vi "YOLO11_OBB_OpenVINO_NIVision.vi"() -> ()   [LabVIEW 2018]
doc: "YOLO11_OBB_OpenVINO_NIVision: This example integrates the YOLO11 algorithm with OpenVINO for object detection with oriented bounding boxes (OBB), specifically using the NI Vision (NIVision) library for enhanced image processing. The combination leverages the power of OpenVINO for optimized inference across Intel hardware and the NI Vision library for advanced vision functions, such as image acquisition, processing, and analysis. The model detects objects in images or video streams and generates oriented bounding boxes (OBB) that provide both the position and rotation of each object, enabling precise localization of rotated or irregularly shaped items. This solution is ideal for real-time industrial or automation applications, where both detection accuracy and processing efficiency are critical. Through the use of OpenVINO and NIVision, the model can run on a variety of platforms, ensuring scalability and performance in diverse environments."
uses:
  vi.lib/VIRobotics/ModelZoo/Object_Detection/yolov8_obb_openvino/Initial_yolo11_Obb_OpenVINO.vi
  vi.lib/VIRobotics/ModelZoo/Object_Detection/yolov8_obb_openvino/yolov8_obb_openvino.lvclass
  <vilib>/vision/driver/NI_Vision_Acquisition_Software.lvlib
panel:
  in  "device_name":string(combo)="CPU"
  in  "class_names_file":path=path "C:/ProgramData/VIRobotics/ModelZoo/Object_Detection/coco.names"
  in  "model_file":path=path "C:/ProgramData/VIRobotics/ModelZoo/Object_Detection/yolo11_obb/onnx_model/yolo11n-obb.onnx"
  in  "Camera Name":refnum<k21>="cam0" caption="IMAQdx Session"
  out "Image":T1(plugin-control)
  in  "Stop":bool
  out "每帧耗时(s)":dbl
  # "Overview: Demonstrates how to use OpenVINO to load the the ONNX model of yolo11_obb for real-time object detection.\nRequirements: Windows.\nMake sure your computer has a camera。\nInstructions: \n1.Select the device_name to use.（If your computer has Intel GPU, you can select GPU in the \"type\" control before running the VI to achieve faster inference).\n2.Run the VI.\nIf you want to load the model you trained, follow the following steps:\n1.Select the device_name to use. \n2.Specify the model_file and class_names_file.\n3.Run the VI."
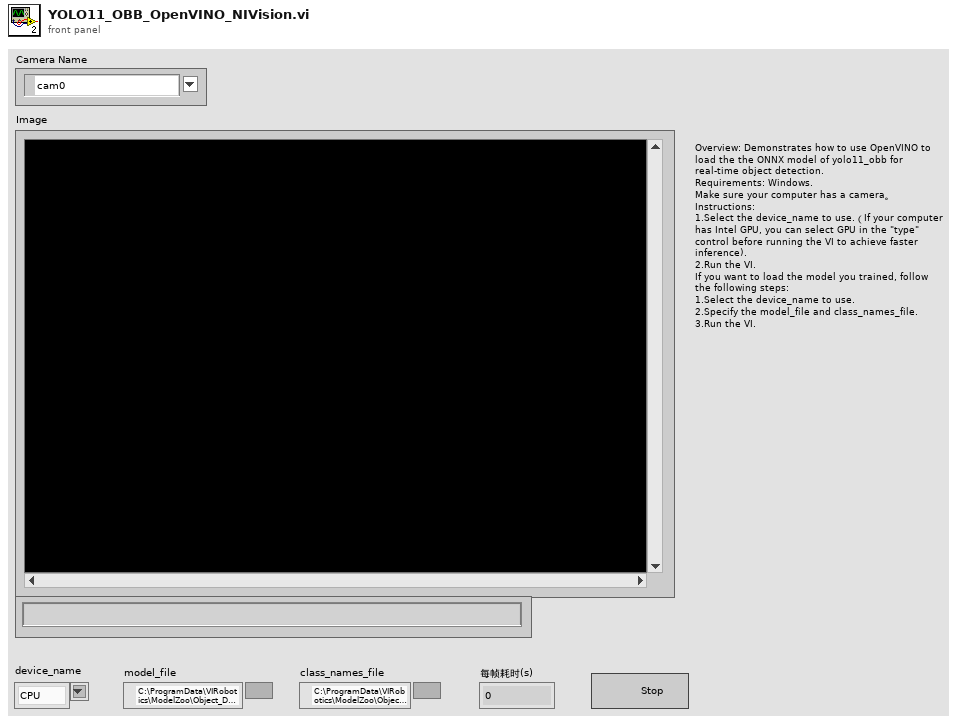
[diagram p1: front panel]
types:
  T1 = typedef "IMAQ Image.ctl" = refnum<image>
  T2 = typedef "IMAQdx.ctl" = refnum<k21>
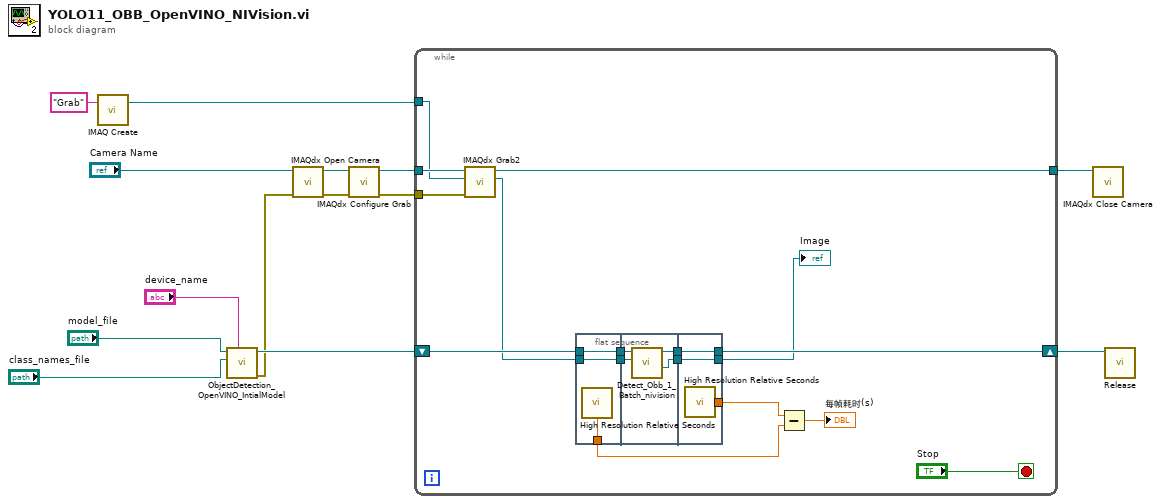
[diagram p0: block diagram]
diagram:
  n1 = call "IMAQ Create"("Image Name"="Grab") -> ("New Image"=w7:T1)  [unwired: 3 in, 2 out]
  n2 = call-poly "ObjectDetection_OpenVINO_IntialModel.vi"("device_name"="device_name", "class_names_path"="class_names_file", "path"="model_file") -> ("error out"=w4:errorcluster, "yolov8_obb_ov out"=w13:refnum<class "yolov8_obb_openvino.lvclass">)  [unwired: 7 in]
  n3 = call <vilib>:"IMAQdx Open Camera.vi"("error in"=w4, "Session In"="Camera Name") -> ("error out"=w12:errorcluster, "Session Out"=w11:T2)  [unwired: 1 in, 7 out]
  n4 = call <vilib>:"IMAQdx Configure Grab.vi"("error in"=w12, "Session In"=w11) -> ("error out"=w5:errorcluster, "Session Out"=w8:T2)  [unwired: 8 out]
  n5 = while {
    shift-right: [w29] -> w14
    shift-left: w13 -> [w30]
    tunnel: w8 -> [w28]
    tunnel: w7 -> [w26]
    tunnel: [w25] -> w6
    tunnel: w5 -> [w24]
    stop <- "Stop" stop-if-true
    n6 = call <vilib>:"IMAQdx Grab2.vi"("error in"=w24, "Image In"=w26, "Session In"=w28) -> ("Image Out"=w23:T1, "Session Out"=w25:T2)  [unwired: 5 in, 2 out]
    n7 = flat-sequence {
      tunnel: w23 -> [w32]
      tunnel: w30 -> [w33]
      tunnel: [w33] -> w19
      tunnel: [w32] -> w18
      tunnel: [w31] -> w17
      tunnel: [w35] -> w21
      tunnel: [w34] -> w20
      tunnel: w19 -> [w37]
      tunnel: w18 -> [w36]
      tunnel: [w39] -> w27
      tunnel: [w40] -> w29
      tunnel: w21 -> [w40]
      tunnel: w20 -> [w39]
      tunnel: [w38] -> w16
      frame #0 {
        n8 = call <vilib>:"High Resolution Relative Seconds.vi"() -> ("relative seconds"=w31:dbl)
      }
      frame #1 {
        n9 = call-dynamic "Detect_Obb_1_Batch_nivision.vi"("Image"=w36, "yolov8_obb_openvino in"=w37) -> ("Image out"=w34:T1, "yolov8_obb_openvino out"=w35:refnum<class "yolov8_obb_openvino.lvclass">)  [unwired: 6 in, 2 out]
      }
      frame #2 {
        n10 = call <vilib>:"High Resolution Relative Seconds.vi"() -> ("relative seconds"=w38:dbl)
      }
    }
    n11 = Subtract(x=w16, y=w17) -> (x-y=→"每帧耗时(s)":dbl)
    "Image" <- w27
  }
  n12 = call <vilib>:"IMAQdx Close Camera.vi"("Session In"=w6) -> ()  [unwired: 1 in, 10 out]
  n13 = call-dynamic "Release.vi"("yolov8_obb_openvino in"=w14) -> ()  [unwired: 9 in, 2 out]
